vi "Main Process.vi"(8 "error in (no error)":errorcluster, 10 "Stop Event":refnum<user-event>, 11 "Service in":refnum<class "Service.lvclass">) -> (0 "error out":errorcluster, 3 "Service out":refnum<class "Service.lvclass">)   [LabVIEW 2024, in "Ramses Framework.lvlib" / "Service.lvclass"]
uses:
  Service.lvclass
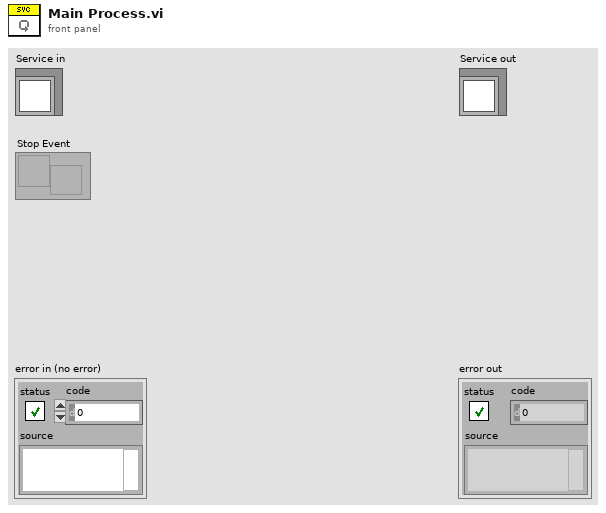
[diagram p1: front panel]
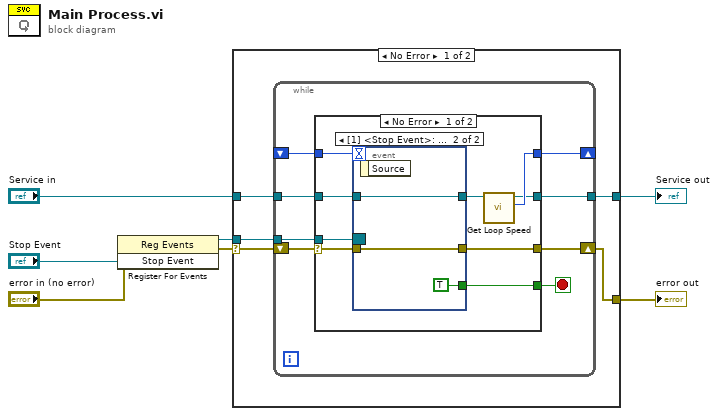
[diagram p0: block diagram]
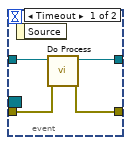
[diagram p2: hidden frame]
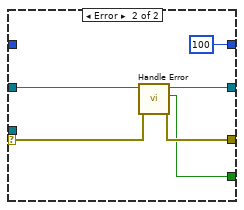
[diagram p3: hidden frame]
diagram:
  n1 = register-events(error in="error in (no error)", "Stop Event") -> (reference out=w4:refnum<event-registration>, error out=w5:errorcluster)  [unwired: 1 in]
  n2 = case shown="No Error" w5 {
    selector: w5 -> [w11 w44]
    tunnel: w4 -> [w12 _]
    tunnel: [w8 w44] -> w3
    tunnel: "Service in" -> [w10 w43]
    tunnel: [w9 w43] -> w1
    frame No Error {
      n3 = while {
        tunnel: w12 -> [w19]
        shift-right: [w13] -> w8
        shift-left: w11 -> [w20]
        shift-right: [w15] -> _
        shift-left: _ -> [w18]
        tunnel: w10 -> [w17]
        tunnel: [w14] -> w9
        stop <- w16 stop-if-true
        n4 = case shown="No Error" w20 {
          selector: w20 -> [w23 w38]
          tunnel: w19 -> [w29 _]
          tunnel: w18 -> [w28 _]
          tunnel: w17 -> [w27 w41]
          tunnel: [w21 w37] -> w16
          tunnel: [w25 100 ("Loop Speed")] -> w15
          tunnel: [w24 w40] -> w14
          tunnel: [w22 w39] -> w13
          frame No Error {
            n5 = event shown="[1] <Stop Event>: User Event" {
              selector: w29 -> [_ _]
              dyn-events: _ -> [_ _]
              timeout: w28 -> [_ _]
              tunnel: [_ TRUE] -> w21
              tunnel: w27 -> [w33 w35]
              tunnel: [w32 w35] -> w26
              tunnel: w23 -> [w30 w34]
              tunnel: [w31 w34] -> w22
              event Timeout {
                n6 = event-data() -> ()  [unwired: 1 in, 1 out]
                n7 = call-dynamic "Do Process.vi"("error in (no error)"=w30, "Service in"=w33) -> ("error out"=w31:errorcluster, "Service out"=w32:refnum<class "Service.lvclass">)  [unwired: 8 in]
              }
              event User Event {
                n8 = event-data() -> ()  [unwired: 1 in, 1 out]
              }
            }
            n9 = call "Get Loop Speed.vi"("Service in"=w26) -> ("Loop Speed"=w25:i32, "Service out"=w24:refnum<class "Service.lvclass">)  [unwired: 8 in, 1 out]
          }
          frame Error {
            n10 = call-dynamic "Handle Error.vi"("error in (no error)"=w38, "Service in"=w41) -> ("error out"=w39:errorcluster, "Stop Process"=w37:bool, "Service out"=w40:refnum<class "Service.lvclass">)  [unwired: 7 in]
          }
        }
      }
    }
    frame Error {
    }
  }
  "error out" <- w3
  "Service out" <- w1
